vi "Generate Log String.vi"(8 "error in (no error)":errorcluster, 11 "ConsoleView Sink in":refnum<class "ConsoleView.lvclass">) -> (0 "error out":errorcluster, 3 "ConsoleView Sink out":refnum<class "ConsoleView.lvclass">, 4 "Log String":string)   [LabVIEW 2017, in "ConsoleView.lvlib" / "ConsoleView.lvclass"]
uses:
  ConsoleView.lvclass
  ConsoleView.lvclass/ConsoleView.ctl
  Filters/Compound Filter/Compound Filter.lvclass
  IStringFormat/IStringFormat.lvclass
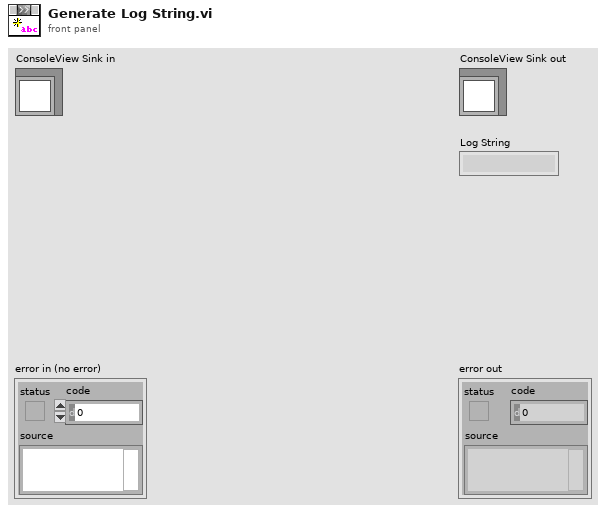
[diagram p1: front panel]
types:
  T1 = typedef "Composed Log.lvlib/Log Packet.ctl" = cluster{"Data To Log":string, "Source":string, "Event Level":T2, "Event Time":timestamp}
  T2 = typedef "Composed Log.lvlib/Log Level.ctl" = enum16{"Debug", "Info", "Warning", "Error", "Critical"}
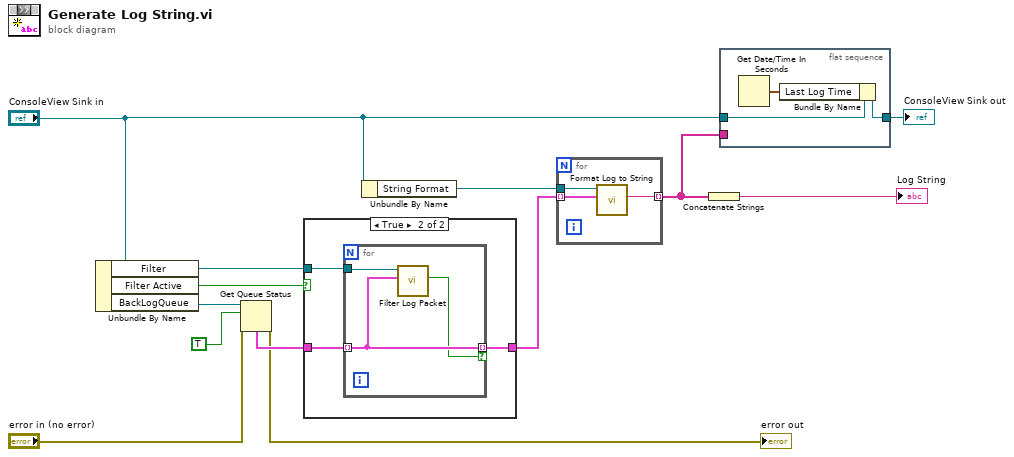
[diagram p0: block diagram]
diagram:
  n1 = Unbundle By Name("ConsoleView Sink in") -> ("Filter"=w9:refnum<class "Compound Filter.lvclass">, "Filter Active"=w10:bool, "BackLogQueue"=w13:refnum<queue>)
  n2 = Get Queue Status(queue=w13, return elements? (F)=TRUE, error in (no error)="error in (no error)") -> (error out=→"error out":errorcluster, elements=w11:T1[])  [unwired: 6 out]
  n3 = case shown="True" w10 {
    tunnel: w11 -> [w14 w16]
    tunnel: w9 -> [_ w17]
    tunnel: [w14 w15] -> w8
    frame False {
    }
    frame True {
      n4 = for {
        tunnel: w17 -> [w20]
        tunnel: w16 -> [w19] mode=indexing
        tunnel: [w19] -> w15 mode=indexing if=w18
        n5 = call-dynamic "Filter Log Packet.vi"("Log Packet"=w19, "Compound Filter in"=w20) -> ("Log?"=w18:bool)  [unwired: 8 in, 1 out]
      }
    }
  }
  n6 = Unbundle By Name("ConsoleView Sink in") -> ("String Format"=w3:refnum<class "IStringFormat.lvclass">)
  n7 = for {
    tunnel: w8 -> [w23] mode=indexing
    tunnel: [w22] -> w1 mode=indexing
    tunnel: w3 -> [w21]
    n8 = call-dynamic "Format Log to String.vi"("Log Packet"=w23, "IStringFormat in"=w21) -> ("Log Entry"=w22:string)  [unwired: 8 in, 1 out]
  }
  n9 = Concatenate Strings(w1) -> (→"Log String":string)
  n10 = flat-sequence {
    tunnel: "ConsoleView Sink in" -> [w26]
    tunnel: [w25] -> w2
    tunnel: w1 -> [_]
    frame #0 {
      n11 = Get Date/Time In Seconds() -> (seconds since 1Jan1904=w24:timestamp)
      n12 = Bundle By Name(cluster=w26, "Last Log Time"=w24) -> (w25:refnum<class "ConsoleView.lvclass">)
    }
  }
  "ConsoleView Sink out" <- w2
